vi "LogDeploymentFailures.vi"(7 "UpdatedDevices":path=path "C:/Users/Public/BatchDeployer/UpdatedDevice.txt", 9 "Names":string[](array[string])) -> ()   [LabVIEW 2016]
panel:
  out "JSON string":string
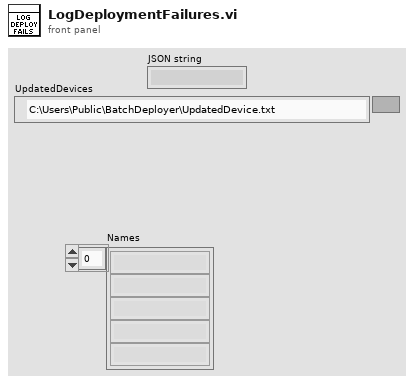
[diagram p1: front panel]
types:
  T1 = enum16{"open", "replace", "create", "open or create", "replace or create", "replace or create with confirmation"}
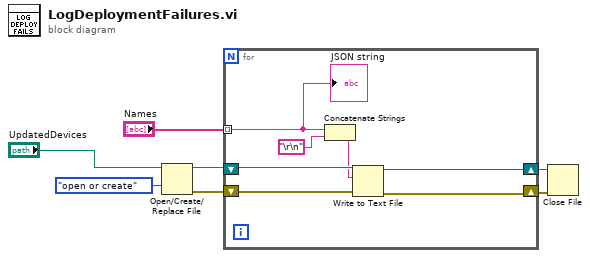
[diagram p0: block diagram]
diagram:
  n1 = Open/Create/Replace File(file path (use dialog)="UpdatedDevices", operation (0:open)=T1."open or create") -> (refnum out=w6:refnum<file>, error out=w4:errorcluster)  [unwired: 4 in, 1 out]
  n2 = for {
    tunnel: "Names" -> [w8] mode=indexing
    shift-right: [w13] -> w5
    shift-left: w6 -> [w14]
    shift-right: [w11] -> w3
    shift-left: w4 -> [w12]
    n3 = Concatenate Strings(w8, "\r\n") -> (w9:string)
    n4 = Write to Text File(file (use dialog)=w14, text=w9, error in=w12) -> (refnum out=w13:refnum<file>, error out=w11:errorcluster)  [unwired: 1 in, 1 out]
    "JSON string" <- w8
  }
  n5 = Close File(refnum=w5, error in=w3) -> ()  [unwired: 2 out]
